vi "UpdateWaferImg.vi"(2 "error in (no error)":errorcluster, 3 "Enum":enum16{"Mark", "Clear All"}(ring), 4 "Wrapper In":refnum<class "EpiWrapper.lvclass">) -> (0 "error out":errorcluster, 1 "Wrapper Out":refnum<class "EpiWrapper.lvclass">)   [LabVIEW 2012]
uses:
  Classes/EpiWrapper.lvclass
  Classes/EpiWrapper.lvclass/EpiWrapper.ctl
  Classes/Get_MeasControl.vi
  Classes/Get_WaferImg.vi
  Classes/Get_MapPOS.vi
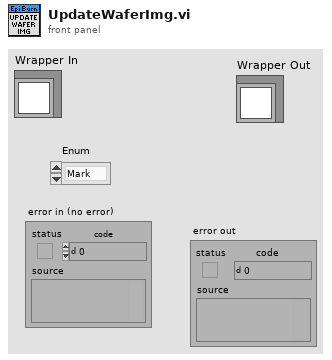
[diagram p1: front panel]
types:
  T1 = cluster{"Width":i16, "Style":enum32{"Solid", "Dash", "Dot", "DashDot", "DashDotDot"}}
  T2 = typedef "MeasureControl.ctl" = cluster{"Pass":bool, "Fail":bool, "Measure":bool, "Area":T3, "TestData":T4, "Graph":cluster{"Y":dbl[], "Y":dbl[]}[]}
  T3 = typedef "TestArea.ctl" = string
  T4 = typedef "TestData.ctl" = cluster{"20mA Data":cluster{"Area":string, "Current,mA":dbl, "Power":dbl, "WL":dbl, "Voltage":dbl, "Knee Current":dbl, "Reverse":dbl}, "50mA Data":cluster{"Area":string, "Current,mA":dbl, "Power":dbl, "WL":dbl, "Voltage":dbl}}
  T5 = typedef "MapPOS.ctl" = cluster{"Top":cluster{"left":i16, "top":i16, "right":i16, "bottom":i16}, "CenterC":cluster{"left":i16, "top":i16, "right":i16, "bottom":i16}, "CenterB":cluster{"left":i16, "top":i16, "right":i16, "bottom":i16}, "CenterA":cluster{"left":i16, "top":i16, "right":i16, "bottom":i16}, "Left":cluster{"left":i16, "top":i16, "right":i16, "bottom":i16}, "Right":cluster{"left":i16, "top":i16, "right":i16, "bottom":i16}}
  T6 = cluster{"left":i16, "top":i16, "right":i16, "bottom":i16}[]
  T7 = typedef "Waferimage.ctl" = picture
  T8 = cluster{"left":i16, "top":i16, "right":i16, "bottom":i16}
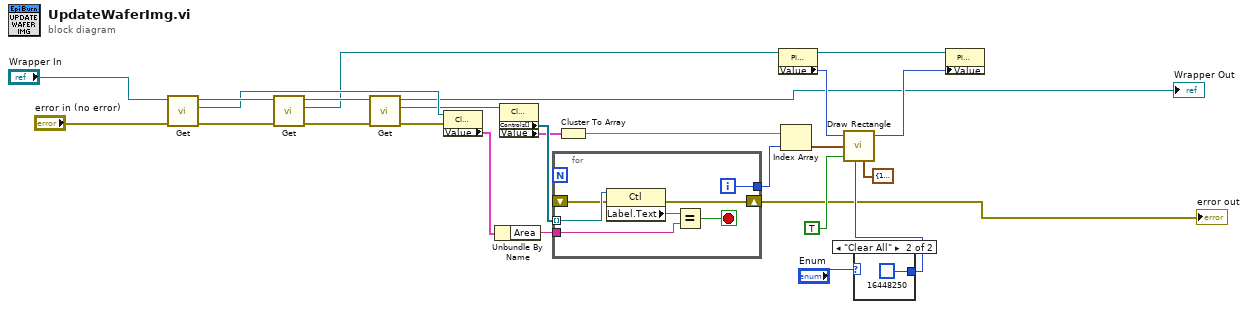
[diagram p0: block diagram]
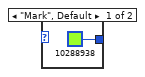
[diagram p2: hidden frame]
diagram:
  n1 = call-poly "Get.vi"("error in (no error)"="error in (no error)", "FrontPanelData in"="Wrapper In") -> ("error out"=w3:errorcluster, "MeasureControl"=w8:refnum<vi>, "FrontPanelData out"=w10:refnum<class "EpiWrapper.lvclass">)  [unwired: 7 in]
  n2 = call-poly "Get.vi"("error in (no error)"=w3, "FrontPanelData in"=w10) -> ("error out"=w4:errorcluster, "Wafer"=w7:refnum<vi>, "FrontPanelData out"=w9:refnum<class "EpiWrapper.lvclass">)  [unwired: 7 in]
  n3 = call-poly "Get.vi"("error in (no error)"=w4, "FrontPanelData in"=w9) -> ("error out"=w5:errorcluster, "MapPOS"=w6:refnum<vi>, "FrontPanelData out"=→"Wrapper Out":refnum<class "EpiWrapper.lvclass">)  [unwired: 7 in]
  n4 = property class="Clust (strict)"(reference=w8, error in=w5) -> ("Value"=w13:T2)  [unwired: 2 out]
  n5 = Unbundle By Name(w13) -> ("Area"=w12:T3)
  n6 = property class="Clust (strict)"(reference=w6) -> ("Controls[]"=w25:refnum<vi>[], "Value"=w18:T5)  [unwired: 1 in, 2 out]
  n7 = for {
    tunnel: w25 -> [w33] mode=indexing
    tunnel: [w30] -> w24
    shift-right: [w28] -> w17
    shift-left: _ -> [w29]
    tunnel: w12 -> [w27]
    i -> [w30]
    stop <- w31 stop-if-true
    n8 = property class="Ctl"(reference=w33, error in=w29) -> (error out=w28:errorcluster, "Label.Text"=w32:string)  [unwired: 1 out]
    n9 = Equal?(x=w32, y=w27) -> (x = y?=w31:bool)
  }
  "error out" <- w17
  n10 = Cluster To Array(cluster=w18) -> (array=w23:T6)
  n11 = property class="Pict (strict)"(reference=w7) -> (reference out=w15:refnum<vi>, "Value"=w16:T7)  [unwired: 1 in, 1 out]
  n12 = Index Array(array=w23, index=w24) -> (element=w22:T8)
  n13 = case shown="\"Clear All\"" "Enum" {
    tunnel: [u32 10288938 ("color(black)") u32 16448250 ("color(black)")] -> w21
    frame "Mark", Default {
    }
    frame "Clear All" {
    }
  }
  n14 = call <vilib>:"Draw Rectangle.vi"("picture"=w16, "rect"=w22, "fill?(F)"=TRUE, "color(black)"=w21, "pen"=T1 {"Width"=1, "Style"=enum."Solid"}) -> ("new picture"=w14:picture)  [unwired: 4 in]
  n15 = property class="Pict (strict)"(reference=w15, "Value"=w14) -> ()  [unwired: 1 in, 2 out]
